vi "Main Page.vi"(8 "error in (no error)":errorcluster, 11 "Node Ptr":T2 format="%.0x") -> (0 "error out":errorcluster)   [LabVIEW 2019, in "Instrument Addon System Explorer.lvlib"]
uses:
  Instrument Addon System Explorer.lvlib
  <vilib>/NI VeriStand/Custom Device API/Custom Device Item Ref.ctl
  Shared/Types/FG Control.ctl
  <vilib>/NI/NI VeriStand Hardware Resource Discovery/Types/Filter Type.ctl
  Shared/Constants.vi
  <vilib>/NI VeriStand/Custom Device API/NI VeriStand - Get Item Property.vi
  <vilib>/NI VeriStand/Custom Device API/Get Item Property (U32).vi
  <vilib>/NI VeriStand/Custom Device API/NI VeriStand - Set Item Property.vi
  <vilib>/NI VeriStand/Custom Device API/Set Item Property (U32).vi
  <vilib>/NI VeriStand/Custom Device API/Get Item Property (String).vi
  <vilib>/NI VeriStand/Custom Device API/Set Item Property (String).vi
  <vilib>/NI VeriStand/Custom Device API/Get Item Property (Boolean).vi
  <vilib>/NI VeriStand/Custom Device API/Set Item Property (Boolean).vi
  <vilib>/Utility/LVClass/Get LV Class Default Value.vi
  Protocols.lvlibp/Protocol Parent/Protocol Parent.lvclass
  <vilib>/NI VeriStand/Custom Device API/Custom Device API.lvlib
  Shared/Instrument Addon Shared.lvlib
  <vilib>/NI/NI VeriStand Hardware Resource Discovery/NIVS Hardware Discovery.lvlib
panel:
  in  "PCL Decimation":u32=1 min=1 max=10000 step=1
  in  "Protocol Settings":enum32{"RS232", "VISA", "TCP/IP", "UDP"}(tab)=enum."VISA"
  in  "COM Browse":bool
  in  "Termination Character":u8=10 format="%.0x"
  in  "End Write":bool=TRUE caption="End Write on Termination Character?"
  in  "End Read":bool=TRUE caption="End Read on Termination Character?"
  in  "XOFF":T1(ring)=enum."DC3"
  in  "XON":T1(ring)=enum."DC1"
  in  "Flow Control":u16(ring) items=["None"=0, "XON/XOFF"=1, "RTS/CTS"=2, "DTR/DSR"=4]
  in  "Stop Bits":u16(ring)=10 items=["1.0"=10, "1.5"=15, "2.0"=20]
  in  "Parity":enum16{"None", "Odd", "Even", "Mark", "Space"}(ring)
  in  "Data Bits":u16=8 min=5 max=8 step=1
  in  "Baud Rate":u32(ring)=9600 items=["75"=75, "110"=110, "134"=134, "150"=150, "300"=300, "600"=600, "1200"=1200, "1800"=1800, "2400"=2400, "4800"=4800, "7200"=7200, "9600"=9600, "14400"=14400, "19200"=19200, "28800"=28800, "38400"=38400, "56000"=56000, "57600"=57600, "115200"=115200, "128000"=128000, "230400"=230400, "460800"=460800, "921600"=921600, "1843200"=1843200, "3000000"=3000000]
  in  "Port":string="COM1"
  in  "VISA Browse":bool
  in  "Append Write Termination Character":bool caption="End Write on Termination Character?"
  in  "Timeout":u32=2000 caption="Timeout (ms)"
  in  "Termination Character":u8=10 format="%.0x"
  in  "Enable Termination Character":bool=TRUE caption="Enable Termination Character?"
  in  "VISA Resource":string="GPIB0::2::INSTR"
  in  "Port":u16
  in  "IP Address":string="localhost"
  in  "UDP Browse":bool
  in  "Target Port":u16
  in  "Target IP Address":string="localhost"
  in  "Local Port":u16
  in  "Local IP Address":string="localhost"
  in  "Protocol":string(combo)
  in  "SHDocVw.IWebBrowser":refnum<k7>(container)
  in  "Header":cluster{"Section Name":string}={"Section Name"="Custom Device Item Settings"}
  in  "Description":string
  in  "Name":string
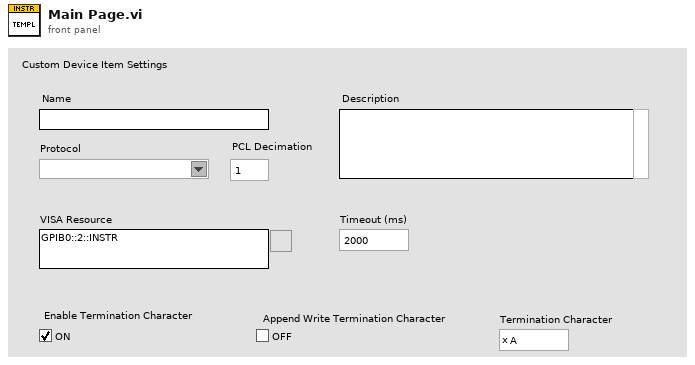
[diagram p1: front panel]
types:
  T1 = enum16{"NUL", "SOH", "STX", "ETX", "EOT", "ENQ", "ACK", "BEL", "BS", "HT", "LF", "VT", "FF", "CR", "SO", "SI", "DLE", "DC1", "DC2", "DC3", "DC4", "NAK", "SYN", "ETB", "CAN", "EM", "SUB", "ESC", "FS", "GS", "RS", "US", "SP", "!", "\"", "#", "$", "%", "&", "'", "(", ")", "*", "+", ",", "- (-)", ".", "/", "0", "1", "2", "3", "4", "5", "6", "7", "8", "9", ":", ";", "<", "=", ">", "?", "@", "A", "B", "C", "D", "E", "F", "G", "H", "I", "J", "K", "L", "M", "N", "O", "P", "Q", "R", "S", "T", "U", "V", "W", "X", "Y", "Z", "[", "\\", "]", "^", "_", "`", "a", "b", "c", "d", "e", "f", "g", "h", "i", "j", "k", "l", "m", "n", "o", "p", "q", "r", "s", "t", "u", "v", "w", "x", "y", "z", "{", "|", "}", "~"}
  T2 = typedef "Custom Device API.lvlib/Custom Device Item Ref.ctl" = u64
  T3 = typedef "Instrument Addon Shared.lvlib/FG Control.ctl" = enum16{"Get", "Set"}
  T4 = typedef "Custom Device API.lvlib/Custom Device Item Info.ctl" = cluster{"Name":string, "Is Channel":bool, "GUID":string, "Is Waveform":bool}
  T5 = typedef "NIVS Hardware Discovery.lvlib/Filter Type.ctl" = enum16{"Device Category", "Product Name", "Ethernet", "XNET", "VISA", "FPGA", "EtherCAT Master", "DAQmx", "GPIB", "Serial"}
  T6 = typedef "Custom Device API.lvlib/Custom Device Commands.ctl" = enum16{"Default", "Item renamed", "Shutdown", "Dynamic button pressed"}
  T7 = typedef "Instrument Addon Shared.lvlib/VISA Settings.ctl" = cluster{"VISA Resource":string, "Enable Termination Character":bool, "Termination Character":u8, "Timeout":u32, "Append Write Termination Character":bool}
  T8 = typedef "Instrument Addon Shared.lvlib/TCPIP Settings.ctl" = cluster{"IP Address":string, "Port":u16}
  T9 = typedef "Instrument Addon Shared.lvlib/UDP Settings.ctl" = cluster{"Local IP Address":string, "Local Port":u16, "Target IP Address":string, "Target Port":u16}
  T10 = typedef "Instrument Addon Shared.lvlib/RSXXX Port Settings.ctl" = cluster{"Port":string, "Baud Rate":u32, "Data Bits":u16, "Parity":enum16{"None", "Odd", "Even", "Mark", "Space"}, "Stop Bits":u16, "Flow Control":u16, "XON":enum16{"NUL", "SOH", "STX", "ETX", "EOT", "ENQ", "ACK", "BEL", "BS", "HT", "LF", "VT", "FF", "CR", "SO", "SI", "DLE", "DC1", "DC2", "DC3", "DC4", "NAK", "SYN", "ETB", "CAN", "EM", "SUB", "ESC", "FS", "GS", "RS", "US", "SP", "!", "\"", "#", "$", "%", "&", "'", "(", ")", "*", "+", ",", "- (-)", ".", "/", "0", "1", "2", "3", "4", "5", "6", "7", "8", "9", ":", ";", "<", "=", ">", "?", "@", "A", "B", "C", "D", "E", "F", "G", "H", "I", "J", "K", "L", "M", "N", "O", "P", "Q", "R", "S", "T", "U", "V", "W", "X", "Y", "Z", "[", "\\", "]", "^", "_", "`", "a", "b", "c", "d", "e", "f", "g", "h", "i", "j", "k", "l", "m", "n", "o", "p", "q", "r", "s", "t", "u", "v", "w", "x", "y", "z", "{", "|", "}", "~"}, "XOFF":enum16{"NUL", "SOH", "STX", "ETX", "EOT", "ENQ", "ACK", "BEL", "BS", "HT", "LF", "VT", "FF", "CR", "SO", "SI", "DLE", "DC1", "DC2", "DC3", "DC4", "NAK", "SYN", "ETB", "CAN", "EM", "SUB", "ESC", "FS", "GS", "RS", "US", "SP", "!", "\"", "#", "$", "%", "&", "'", "(", ")", "*", "+", ",", "- (-)", ".", "/", "0", "1", "2", "3", "4", "5", "6", "7", "8", "9", ":", ";", "<", "=", ">", "?", "@", "A", "B", "C", "D", "E", "F", "G", "H", "I", "J", "K", "L", "M", "N", "O", "P", "Q", "R", "S", "T", "U", "V", "W", "X", "Y", "Z", "[", "\\", "]", "^", "_", "`", "a", "b", "c", "d", "e", "f", "g", "h", "i", "j", "k", "l", "m", "n", "o", "p", "q", "r", "s", "t", "u", "v", "w", "x", "y", "z", "{", "|", "}", "~"}, "End Read on Termination Character":bool, "End Write on Termination Character":bool, "Termination Character":u8}
  T11 = typedef "Protocols.lvlibp/Protocol Parent.lvclass/Base Protocol Type.ctl" = enum16{"RS-XXX", "VISA", "TCPIP", "UDP"}
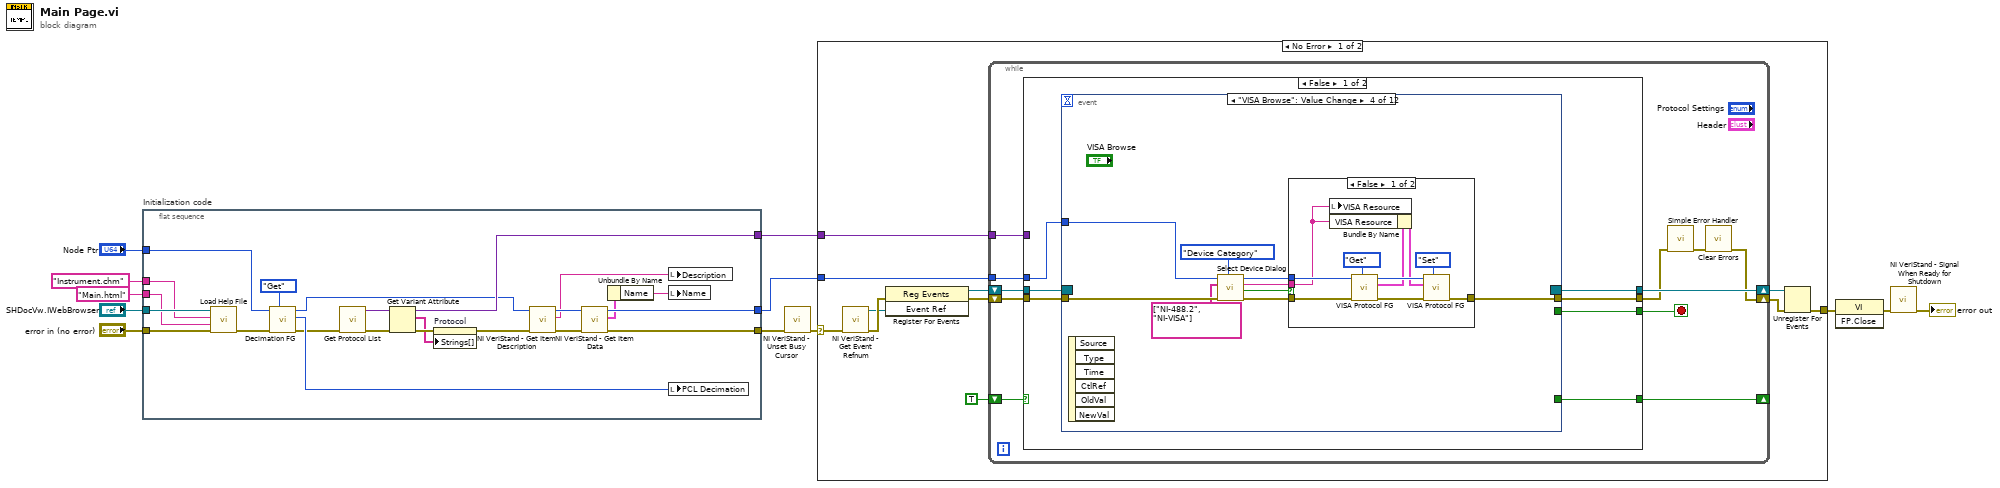
[diagram p0: block diagram]
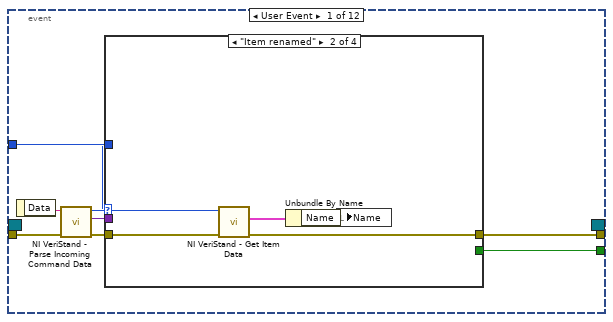
[diagram p2: hidden frame]
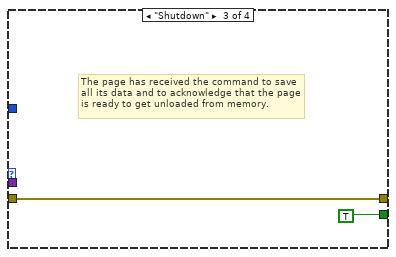
[diagram p4: hidden frame]
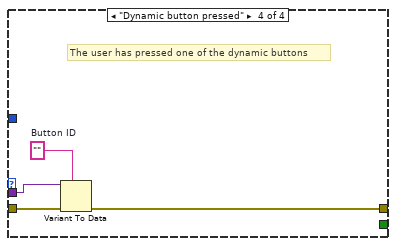
[diagram p5: hidden frame]
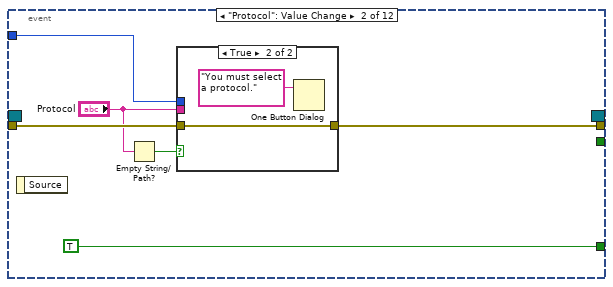
[diagram p6: hidden frame]
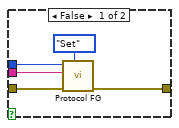
[diagram p7: hidden frame]
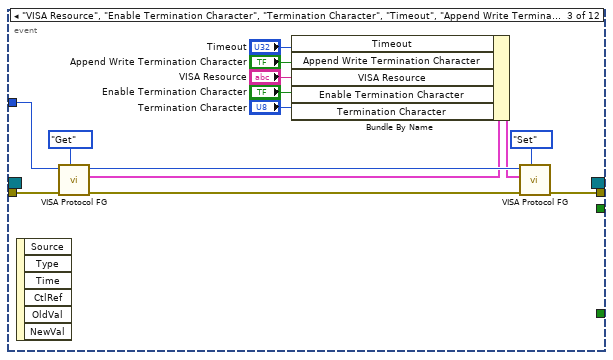
[diagram p8: hidden frame]
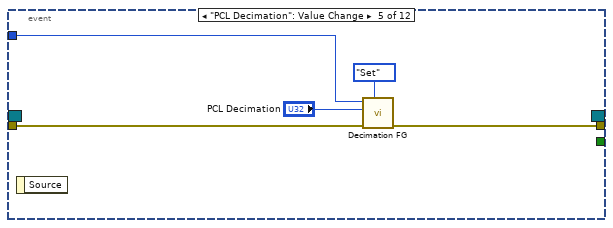
[diagram p10: hidden frame]
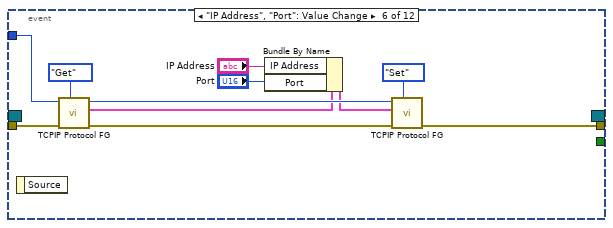
[diagram p11: hidden frame]
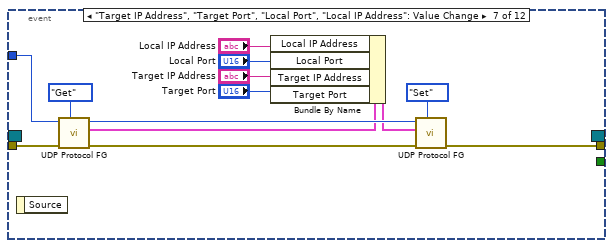
[diagram p12: hidden frame]
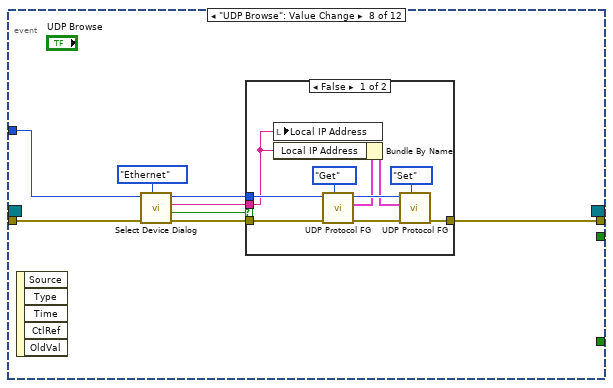
[diagram p13: hidden frame]
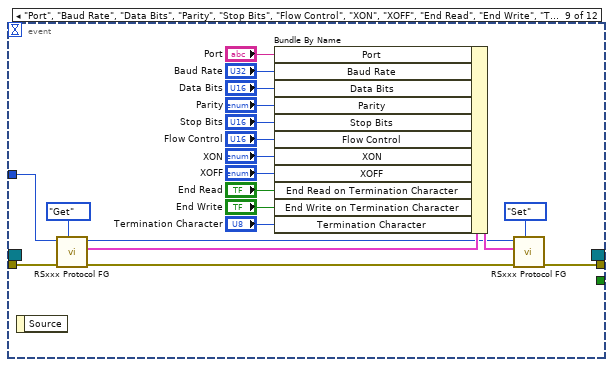
[diagram p15: hidden frame]
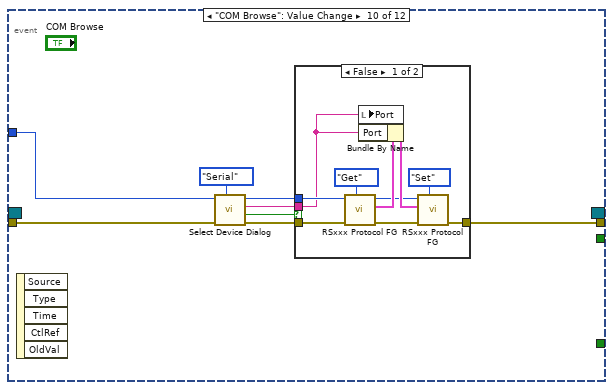
[diagram p16: hidden frame]
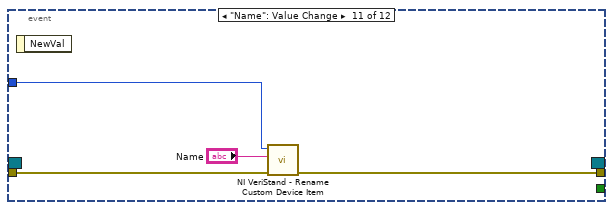
[diagram p18: hidden frame]
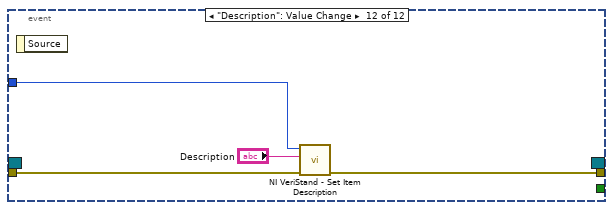
[diagram p19: hidden frame]
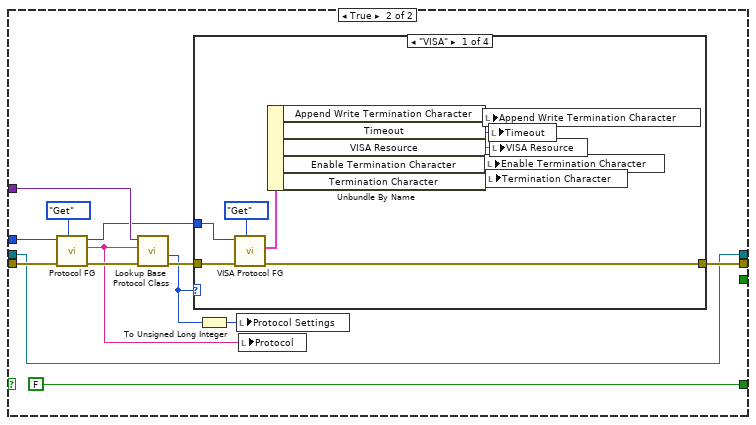
[diagram p20: hidden frame]
diagram:
  n1 = flat-sequence "Initialization code" {
    tunnel: "error in (no error)" -> [w28]
    tunnel: "Node Ptr" -> [w24]
    tunnel: [w29] -> w8
    tunnel: [w35] -> w5
    tunnel: "SHDocVw.IWebBrowser" -> [w27]
    tunnel: "Main.html" ("HTML File") -> [w26]
    tunnel: "Instrument.chm" ("Main CHM File") -> [w25]
    tunnel: [w16] -> w1
    frame #0 {
      n2 = call "Load Help File.vi"("error in (no error)"=w28, "HTML File"=w26, "Main CHM File"=w25, "SHDocVw.IWebBrowser2"=w27) -> ("error out"=w23:errorcluster)  [unwired: 7 in]
      n3 = call "Decimation FG.vi"("Action"=FG_Control."Get", "error in (no error)"=w23, "Device Item Ref in"=w24) -> ("error out"=w14:errorcluster, "Decimation out"=w21:u32, "Item Ref out"=w13:T2)  [unwired: 6 in]
      n4 = call "Get Protocol List.vi"("error in (no error)"=w14) -> ("error out"=w19:errorcluster, "Class Lookup"=w20:variant)  [unwired: 9 in]
      n5 = Get Variant Attribute(Variant=w20, error in=w19) -> (duplicate Variant=w16:variant, names=w17:string[], error out=w18:errorcluster)  [unwired: 2 in, 1 out]
      n6 = property on="Protocol" class="CmbBox"(error in=w18, "Strings[]"=w17) -> (error out=w15:errorcluster)  [unwired: 1 in, 1 out]
      n7 = call <vilib>:"NI VeriStand - Get Item Description.vi"("error in (no error)"=w15, "Item Ref in"=w13) -> ("error out"=w32:errorcluster, "Description"=w33:string, "Item Ref out"=w34:T2)  [unwired: 7 out]
      n8 = call <vilib>:"NI VeriStand - Get Item Data.vi"("error in (no error)"=w32, "Item Ref in"=w34) -> ("error out"=w29:errorcluster, "Item Info"=w31:T4, "Item Ref out"=w35:T2)  [unwired: 7 out]
      n9 = Unbundle By Name(w31) -> ("Name"=w30:string)
      n10 = local write "Description"(w33) -> ()
      n11 = local write "Name"(w30) -> ()
      n12 = local write "PCL Decimation"(w21) -> ()
    }
  }
  n13 = call <vilib>:"NI VeriStand - Unset Busy Cursor.vi"("error in (no error)"=w8) -> ("error out"=w7:errorcluster)  [unwired: 10 out]
  n14 = case shown="No Error" w7 {
    selector: w7 -> [w38 w284]
    tunnel: [w43 w282] -> w12
    tunnel: w5 -> [w39 _]
    tunnel: w1 -> [w37 _]
    frame No Error {
      n15 = call <vilib>:"NI VeriStand - Get Event Refnum.vi"("error in (no error)"=w38) -> ("error out"=w46:errorcluster, "Event Ref"=w42:refnum<user-event>)  [unwired: 9 out]
      n16 = register-events(error in=w46, w42) -> (reference out=w40:refnum<event-registration>, error out=w41:errorcluster)  [unwired: 1 in]
      n17 = while {
        tunnel: w39 -> [w53]
        shift-right: [w50] -> w44
        shift-left: w41 -> [w56]
        shift-right: [w57] -> w45
        shift-left: w40 -> [w55]
        tunnel: w37 -> [w49]
        shift-right: [w47] -> _
        shift-left: TRUE -> [w48]
        stop <- w54 stop-if-true
        n18 = case shown="False" w48 {
          tunnel: [w64 w229] -> w57
          tunnel: w56 -> [w63 w238]
          tunnel: w55 -> [w62 w229]
          tunnel: [w61 _] -> w54
          tunnel: w53 -> [w60 w237]
          tunnel: [w59 w230] -> w52
          tunnel: w49 -> [_ w235]
          tunnel: [w58 FALSE] -> w47
          frame False {
            n19 = event shown="[3] \"VISA Browse\": Value Change" {
              selector: w62 -> [_ _ _ _ _ _ _ _ _ _ _ _]
              dyn-events: [_ _ _ _ _ _ _ _ _ _ _ _] -> w64
              timeout: _ -> [_ _ _ _ _ _ _ _ _ _ _ _]
              tunnel: w63 -> [w72 w89 w110 w119 w135 w146 w159 w167 w196 w206 w222 w225]
              tunnel: [w68 _ _ _ _ _ _ _ _ _ _ _] -> w61
              tunnel: [w67 w85 w106 w120 w133 w142 w155 w168 w198 w207 w221 w224] -> w59
              tunnel: w60 -> [w66 w90 w109 w117 w134 w145 w158 w165 w194 w205 w220 w226]
              tunnel: [_ TRUE _ _ _ _ _ _ _ _ _ _] -> w58
              event User Event {
                n20 = event-data() -> ("Data"=w71:string)  [unwired: 1 out]
                n21 = call <vilib>:"NI VeriStand - Parse Incoming Command Data.vi"("error in (no error)"=w72, "Incoming data"=w71) -> ("error out"=w70:errorcluster, "Outgoing data"=w65:variant, "Action"=w69:T6)  [unwired: 7 out]
                n22 = case shown="\"Item renamed\"" w69 {
                  tunnel: w70 -> [w73 w78 w79 w84]
                  tunnel: [_ _ TRUE _] -> w68
                  tunnel: [w73 w75 w79 w81] -> w67
                  tunnel: w66 -> [_ w77 _ _]
                  tunnel: w65 -> [_ _ _ w83]
                  frame "Default", Default {
                  }
                  frame "Item renamed" {
                    n23 = call <vilib>:"NI VeriStand - Get Item Data.vi"("error in (no error)"=w78, "Item Ref in"=w77) -> ("error out"=w75:errorcluster, "Item Info"=w76:T4)  [unwired: 8 out]
                    n24 = Unbundle By Name(w76) -> ("Name"=w74:string)
                    n25 = local write "Name"(w74) -> ()
                  }
                  frame "Shutdown" {
                    # "The page has received the command to save all its data and to acknowledge that the page is ready to get unloaded from memory."
                  }
                  frame "Dynamic button pressed" {
                    w82 = ""  # Button ID
                    # "The user has pressed one of the dynamic buttons"
                    n26 = Variant To Data(error in=w84, type=w82, Variant=w83) -> (error out=w81:errorcluster)  [unwired: 1 out]
                  }
                }
              }
              event "Protocol": Value Change {
                n27 = event-data() -> ()  [unwired: 2 out]
                n28 = Empty String/Path?(string/path="Protocol") -> (empty?=w87:bool)
                n29 = case shown="True" w87 {
                  tunnel: w90 -> [w93 _]
                  tunnel: w89 -> [w94 w96]
                  tunnel: [w91 w96] -> w85
                  tunnel: "Protocol" -> [w92 _]
                  frame False {
                    n30 = call "Protocol FG.vi"("Action"=FG_Control."Set", "error in (no error)"=w94, "Protocol"=w92, "Device Item Ref in"=w93) -> ("error out"=w91:errorcluster)  [unwired: 5 in, 2 out]
                  }
                  frame True {
                    n31 = One Button Dialog(message="You must select a protocol.") -> ()  [unwired: 1 in, 1 out]
                  }
                }
              }
              event "VISA Resource", "Enable Termination Character", "Termination Character", "Timeout", "Append Write Termination Character": Value Change {
                n32 = event-data() -> ()  [unwired: 7 out]
                n33 = call "VISA Protocol FG.vi"("Action"=FG_Control."Get", "error in (no error)"=w110, "Device Item Ref in"=w109) -> ("error out"=w107:errorcluster, "VISA Config"=w104:T7, "Item Ref out"=w105:T2)  [unwired: 6 in]
                n34 = Bundle By Name(cluster=w104, "Timeout"="Timeout", "Append Write Termination Character"="Append Write Termination Character", "VISA Resource"="VISA Resource", "Enable Termination Character"="Enable Termination Character", "Termination Character"="Termination Character") -> (w103:T7)
                n35 = call "VISA Protocol FG.vi"("Action"=FG_Control."Set", "error in (no error)"=w107, "VISA Config"=w103, "Device Item Ref in"=w105) -> ("error out"=w106:errorcluster)  [unwired: 5 in, 2 out]
              }
              event "VISA Browse": Value Change {
                n36 = event-data() -> ()  [unwired: 7 out]
                n37 = call <vilib>:"Select Device Dialog.vi"("Filter Type"=Filter_Type."Device Category", "error in (no error)"=w119, "Filter Names"=string[] ["NI-488.2", "NI-VISA"], "Item Ref in"=w117) -> ("error out"=w118:errorcluster, "Cancelled?"=w115:bool, "Selected Alias"=w114:string, "Item Ref out"=w116:T2)  [unwired: 4 in]
                n38 = case shown="False" w115 {
                  tunnel: w118 -> [w129 w131]
                  tunnel: w116 -> [w128 _]
                  tunnel: [w125 w131] -> w120
                  tunnel: w114 -> [w121 _]
                  frame False {
                    n39 = local write "VISA Resource"(w121) -> ()
                    n40 = call "VISA Protocol FG.vi"("Action"=FG_Control."Get", "error in (no error)"=w129, "Device Item Ref in"=w128) -> ("error out"=w126:errorcluster, "VISA Config"=w123:T7, "Item Ref out"=w124:T2)  [unwired: 6 in]
                    n41 = Bundle By Name(cluster=w123, "VISA Resource"=w121) -> (w122:T7)
                    n42 = call "VISA Protocol FG.vi"("Action"=FG_Control."Set", "error in (no error)"=w126, "VISA Config"=w122, "Device Item Ref in"=w124) -> ("error out"=w125:errorcluster)  [unwired: 5 in, 2 out]
                  }
                  frame True {
                  }
                }
              }
              event "PCL Decimation": Value Change {
                n43 = event-data() -> ()  [unwired: 2 out]
                n44 = call "Decimation FG.vi"("Action"=FG_Control."Set", "error in (no error)"=w135, "Decimation"="PCL Decimation", "Device Item Ref in"=w134) -> ("error out"=w133:errorcluster)  [unwired: 5 in, 2 out]
              }
              event "IP Address", "Port": Value Change {
                n45 = event-data() -> ()  [unwired: 2 out]
                n46 = call "TCPIP Protocol FG.vi"("Action"=FG_Control."Get", "error in (no error)"=w146, "Device Item Ref in"=w145) -> ("error out"=w143:errorcluster, "TCP/IP Config"=w140:T8, "Item Ref out"=w141:T2)  [unwired: 6 in]
                n47 = Bundle By Name(cluster=w140, "IP Address"="IP Address", "Port"="Port") -> (w139:T8)
                n48 = call "TCPIP Protocol FG.vi"("Action"=FG_Control."Set", "error in (no error)"=w143, "TCP/IP Config"=w139, "Device Item Ref in"=w141) -> ("error out"=w142:errorcluster)  [unwired: 5 in, 2 out]
              }
              event "Target IP Address", "Target Port", "Local Port", "Local IP Address": Value Change {
                n49 = event-data() -> ()  [unwired: 2 out]
                n50 = call "UDP Protocol FG.vi"("Action"=FG_Control."Get", "error in (no error)"=w159, "Device Item Ref in"=w158) -> ("error out"=w156:errorcluster, "UDP Config"=w153:T9, "Item Ref out"=w154:T2)  [unwired: 6 in]
                n51 = Bundle By Name(cluster=w153, "Local IP Address"="Local IP Address", "Local Port"="Local Port", "Target IP Address"="Target IP Address", "Target Port"="Target Port") -> (w152:T9)
                n52 = call "UDP Protocol FG.vi"("Action"=FG_Control."Set", "error in (no error)"=w156, "UDP Config"=w152, "Device Item Ref in"=w154) -> ("error out"=w155:errorcluster)  [unwired: 5 in, 2 out]
              }
              event "UDP Browse": Value Change {
                n53 = event-data() -> ()  [unwired: 6 out]
                n54 = call <vilib>:"Select Device Dialog.vi"("Filter Type"=Filter_Type."Ethernet", "error in (no error)"=w167, "Item Ref in"=w165) -> ("error out"=w166:errorcluster, "Cancelled?"=w163:bool, "Selected Alias"=w162:string, "Item Ref out"=w164:T2)  [unwired: 5 in]
                n55 = case shown="False" w163 {
                  tunnel: w166 -> [w177 w179]
                  tunnel: w164 -> [w176 _]
                  tunnel: [w173 w179] -> w168
                  tunnel: w162 -> [w169 _]
                  frame False {
                    n56 = local write "Local IP Address"(w169) -> ()
                    n57 = call "UDP Protocol FG.vi"("Action"=FG_Control."Get", "error in (no error)"=w177, "Device Item Ref in"=w176) -> ("error out"=w174:errorcluster, "UDP Config"=w171:T9, "Item Ref out"=w172:T2)  [unwired: 6 in]
                    n58 = Bundle By Name(cluster=w171, "Local IP Address"=w169) -> (w170:T9)
                    n59 = call "UDP Protocol FG.vi"("Action"=FG_Control."Set", "error in (no error)"=w174, "UDP Config"=w170, "Device Item Ref in"=w172) -> ("error out"=w173:errorcluster)  [unwired: 5 in, 2 out]
                  }
                  frame True {
                  }
                }
              }
              event "Port", "Baud Rate", "Data Bits", "Parity", "Stop Bits", "Flow Control", "XON", "XOFF", "End Read", "End Write", "Termination Character": Value Change {
                n60 = event-data() -> ()  [unwired: 2 out]
                n61 = call "RSxxx Protocol FG.vi"("Action"=FG_Control."Get", "error in (no error)"=w196, "Device Item Ref in"=w194) -> ("error out"=w195:errorcluster, "Serial Config"=w193:T10, "Item Ref out"=w180:T2)  [unwired: 6 in]
                n62 = Bundle By Name(cluster=w193, "Port"="Port", "Baud Rate"="Baud Rate", "Data Bits"="Data Bits", "Parity"="Parity", "Stop Bits"="Stop Bits", "Flow Control"="Flow Control", "XON"="XON", "XOFF"="XOFF", "End Read on Termination Character"="End Read", "End Write on Termination Character"="End Write", "Termination Character"="Termination Character") -> (w192:T10)
                n63 = call "RSxxx Protocol FG.vi"("Action"=FG_Control."Set", "error in (no error)"=w195, "Serial Config"=w192, "Device Item Ref in"=w180) -> ("error out"=w198:errorcluster)  [unwired: 5 in, 2 out]
              }
              event "COM Browse": Value Change {
                n64 = event-data() -> ()  [unwired: 6 out]
                n65 = call <vilib>:"Select Device Dialog.vi"("Filter Type"=Filter_Type."Serial", "error in (no error)"=w206, "Item Ref in"=w205) -> ("error out"=w203:errorcluster, "Cancelled?"=w202:bool, "Selected Alias"=w201:string, "Item Ref out"=w204:T2)  [unwired: 5 in]
                n66 = case shown="False" w202 {
                  tunnel: [w216 w218] -> w207
                  tunnel: w203 -> [w214 w218]
                  tunnel: w204 -> [w212 _]
                  tunnel: w201 -> [w208 _]
                  frame False {
                    n67 = call "RSxxx Protocol FG.vi"("Action"=FG_Control."Get", "error in (no error)"=w214, "Device Item Ref in"=w212) -> ("error out"=w213:errorcluster, "Serial Config"=w211:T10, "Item Ref out"=w209:T2)  [unwired: 6 in]
                    n68 = local write "Port"(w208) -> ()
                    n69 = Bundle By Name(cluster=w211, "Port"=w208) -> (w210:T10)
                    n70 = call "RSxxx Protocol FG.vi"("Action"=FG_Control."Set", "error in (no error)"=w213, "Serial Config"=w210, "Device Item Ref in"=w209) -> ("error out"=w216:errorcluster)  [unwired: 5 in, 2 out]
                  }
                  frame True {
                  }
                }
              }
              event "Name": Value Change {
                n71 = event-data() -> ()  [unwired: 2 out]
                n72 = call <vilib>:"NI VeriStand - Rename Custom Device Item.vi"("error in (no error)"=w222, "New Name"="Name", "Item Ref in"=w220) -> ("error out"=w221:errorcluster)  [unwired: 1 in, 7 out]
              }
              event "Description": Value Change {
                n73 = event-data() -> ()  [unwired: 2 out]
                n74 = call <vilib>:"NI VeriStand - Set Item Description.vi"("error in (no error)"=w225, "Description"="Description", "Item Ref in"=w226) -> ("error out"=w224:errorcluster)  [unwired: 8 out]
              }
            }
          }
          frame True {
            n75 = call "Protocol FG.vi"("Action"=FG_Control."Get", "error in (no error)"=w238, "Device Item Ref in"=w237) -> ("error out"=w234:errorcluster, "Protocol out"=w231:string, "Item Ref out"=w233:T2)  [unwired: 6 in]
            n76 = call "Lookup Base Protocol Class.vi"("error in (no error)"=w234, "Protocol in"=w231, "Class Lookup"=w235) -> ("error out"=w236:errorcluster, "Protocol out"=w228:T11)  [unwired: 5 in, 2 out]
            n77 = case shown="\"VISA\"" w228 {
              tunnel: w236 -> [w249 w256 w265 w281]
              tunnel: [w248 w255 w264 w280] -> w230
              tunnel: w233 -> [w247 w254 w263 w279]
              frame "VISA" {
                n78 = call "VISA Protocol FG.vi"("Action"=FG_Control."Get", "error in (no error)"=w249, "Device Item Ref in"=w247) -> ("error out"=w248:errorcluster, "VISA Config"=w245:T7)  [unwired: 6 in, 1 out]
                n79 = Unbundle By Name(w245) -> ("Append Write Termination Character"=w240:bool, "Timeout"=w241:u32, "VISA Resource"=w244:string, "Enable Termination Character"=w243:bool, "Termination Character"=w242:u8)
                n80 = local write "Append Write Termination Character"(w240) -> ()
                n81 = local write "Enable Termination Character"(w243) -> ()
                n82 = local write "Termination Character"(w242) -> ()
                n83 = local write "Timeout"(w241) -> ()
                n84 = local write "VISA Resource"(w244) -> ()
              }
              frame "TCPIP" {
                n85 = call "TCPIP Protocol FG.vi"("Action"=FG_Control."Get", "error in (no error)"=w256, "Device Item Ref in"=w254) -> ("error out"=w255:errorcluster, "TCP/IP Config"=w252:T8)  [unwired: 6 in, 1 out]
                n86 = Unbundle By Name(w252) -> ("IP Address"=w251:string, "Port"=w250:u16)
                n87 = local write "IP Address"(w251) -> ()
                n88 = local write "Port"(w250) -> ()
              }
              frame "UDP" {
                n89 = call "UDP Protocol FG.vi"("Action"=FG_Control."Get", "error in (no error)"=w265, "Device Item Ref in"=w263) -> ("error out"=w264:errorcluster, "UDP Config"=w261:T9)  [unwired: 6 in, 1 out]
                n90 = Unbundle By Name(w261) -> ("Local IP Address"=w260:string, "Local Port"=w259:u16, "Target IP Address"=w258:string, "Target Port"=w257:u16)
                n91 = local write "Local IP Address"(w260) -> ()
                n92 = local write "Local Port"(w259) -> ()
                n93 = local write "Target IP Address"(w258) -> ()
                n94 = local write "Target Port"(w257) -> ()
              }
              frame "RS-XXX" {
                n95 = call "RSxxx Protocol FG.vi"("Action"=FG_Control."Get", "error in (no error)"=w281, "Device Item Ref in"=w279) -> ("error out"=w280:errorcluster, "Serial Config"=w277:T10)  [unwired: 6 in, 1 out]
                n96 = Unbundle By Name(w277) -> ("Port"=w276:string, "Baud Rate"=w275:u32, "Data Bits"=w266:u16, "Parity"=w267:enum16{"None", "Odd", "Even", "Mark", "Space"}, "Stop Bits"=w268:u16, "Flow Control"=w269:u16, "XON"=w270:T1, "XOFF"=w271:T1, "End Read on Termination Character"=w272:bool, "End Write on Termination Character"=w273:bool, "Termination Character"=w274:u8)
                n97 = local write "Termination Character"(w274) -> ()
                n98 = local write "Flow Control"(w269) -> ()
                n99 = local write "Data Bits"(w266) -> ()
                n100 = local write "Stop Bits"(w268) -> ()
                n101 = local write "XON"(w270) -> ()
                n102 = local write "End Write"(w273) -> ()
                n103 = local write "Port"(w276) -> ()
                n104 = local write "Baud Rate"(w275) -> ()
                n105 = local write "Parity"(w267) -> ()
                n106 = local write "XOFF"(w271) -> ()
                n107 = local write "End Read"(w272) -> ()
              }
            }
            n108 = To Unsigned Long Integer(number=w228) -> (unsigned 32bit integer=w232:u32)
            n109 = local write "Protocol Settings"(w232) -> ()
            n110 = local write "Protocol"(w231) -> ()
          }
        }
        n111 = call <vilib>:"Simple Error Handler.vi"("error in (no error)"=w52) -> ("error out"=w51:errorcluster)  [unwired: 1 in, 7 out]
        n112 = call <vilib>:"Clear Errors.vi"("error in (no error)"=w51) -> ("error out"=w50:errorcluster)  [unwired: 1 in, 5 out]
      }
      n113 = Unregister For Events(event registration refnum=w45, error in=w44) -> (error out=w43:errorcluster)
    }
    frame Error {
      n114 = call <vilib>:"Simple Error Handler.vi"("error in (no error)"=w284) -> ("error out"=w283:errorcluster)  [unwired: 1 in, 7 out]
      n115 = call <vilib>:"Clear Errors.vi"("error in (no error)"=w283) -> ("error out"=w282:errorcluster)  [unwired: 1 in, 5 out]
    }
  }
  n116 = invoke class="VI" method="FP.Close"(error in=w12) -> (error out=w11:errorcluster)  [unwired: 2 in, 2 out]
  n117 = call <vilib>:"NI VeriStand - Signal When Ready for Shutdown.vi"("error in (no error)"=w11) -> ("error out"=→"error out":errorcluster)  [unwired: 10 out]
